vi "Vehicle Constructor.vi"(11 "Vehicle Model":string) -> (0 "error out":errorcluster, 3 "Vehicle.lvclass":refnum<class "Vehicle.lvclass">)   [LabVIEW 2024, in "Vehicle.lvclass"]
uses:
  Vehicle.lvclass
  VehicleModelPlatinum/VehicleModelPlatinum.lvclass
  VehicleModelBase/VehicleModelBase.lvclass
  VehicleModel/VehicleModel.lvclass
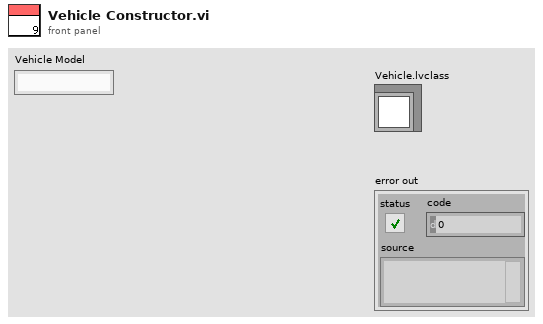
[diagram p1: front panel]
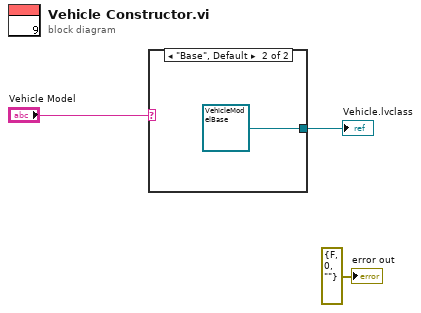
[diagram p0: block diagram]
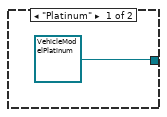
[diagram p2: hidden frame]
diagram:
  n1 = case shown="\"Base\", Default" "Vehicle Model" {
    tunnel: [refnum<class "VehicleModelPlatinum.lvclass"> refnum ("VehicleModelPlatinum.lvclass") refnum<class "VehicleModelBase.lvclass"> refnum ("VehicleModelBase.lvclass")] -> w3
    frame "Platinum" {
    }
    frame "Base", Default {
    }
  }
  "Vehicle.lvclass" <- w3
  "error out" <- errorcluster {"status"=FALSE, "code"=0, "source"=""} ("error out")
